vi "Recursive find VIs.vi"(8 "error in (no error)":errorcluster, 11 "Project Items":refnum<vi>[](array[refnum])) -> (0 "error out":errorcluster, 3 "VIs":set{path}(c389))   [LabVIEW 2020, in "Coverage Report.lvclass"]
uses:
  Coverage Report.lvclass
  a1401d1e-ec1c-4a27-9029-e4c0d22f2509.vi
  Coverage Report.lvclass/Coverage Report.ctl
  <vilib>/Astemes/LUnit/Test Case.lvclass
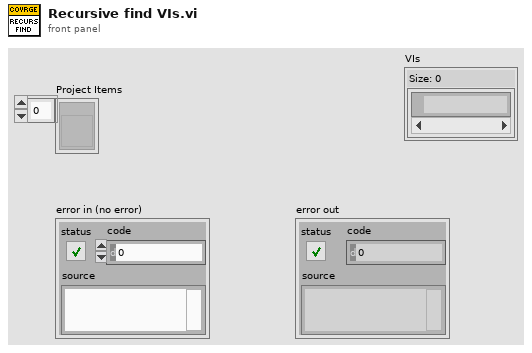
[diagram p1: front panel]
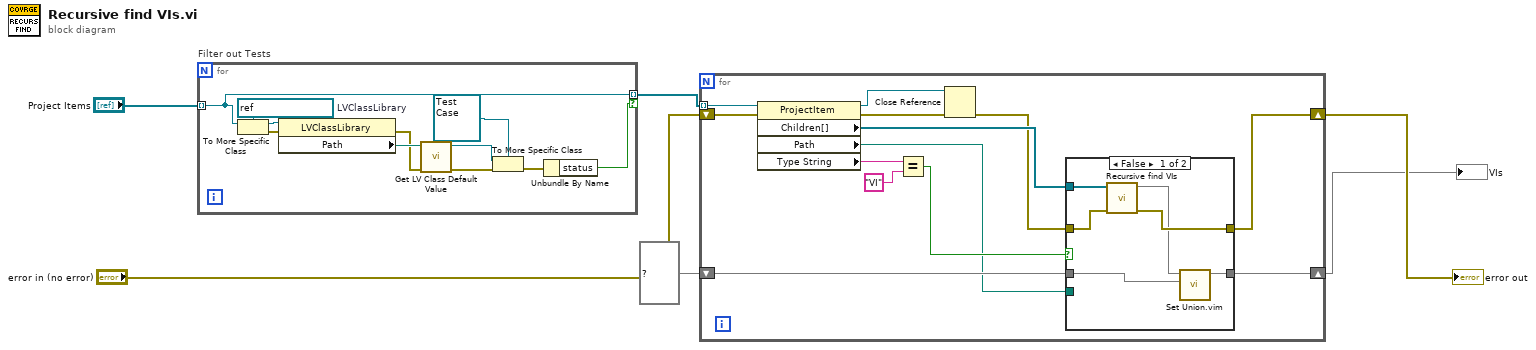
[diagram p0: block diagram]
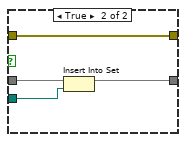
[diagram p2: hidden frame]
diagram:
  n1 = for "Filter out Tests" {
    tunnel: "Project Items" -> [w9] mode=indexing
    tunnel: [w9] -> w1 mode=indexing if=w8
    w17 = refnum<vi> refnum  # LVClassLibrary
    n2 = To More Specific Class(target class=w17, reference=w9) -> (specific class reference=w16:refnum<vi>, error out=w15:errorcluster)  [unwired: 1 in]
    n3 = property class="LVClassLibrary"(reference=w16, error in=w15) -> (error out=w13:errorcluster, "Path"=w14:path)  [unwired: 1 out]
    n4 = call <vilib>:"Get LV Class Default Value.vi"("error in (no error)"=w13, "class path"=w14) -> ("error out"=w12:errorcluster, "object"=w11:refnum<class>)  [unwired: 8 in]
    n5 = To More Specific Class(target class=refnum<class "Test Case.lvclass"> refnum ("LUnit Test Case In"), reference=w11, error in=w12) -> (error out=w10:errorcluster)  [unwired: 1 out]
    n6 = Unbundle By Name(w10) -> ("status"=w8:bool)
  }
  n7 = for {
    tunnel: w1 -> [w27] mode=indexing
    shift-right: [w21] -> w6
    shift-left: "error in (no error)" -> [w26]
    shift-right: [w19] -> w4
    shift-left: set{path} {} ("VIs") -> [w20]
    n8 = property class="ProjectItem"(reference=w27, error in=w26) -> (reference out=w24:refnum<vi>, error out=w25:errorcluster, "Children[]"=w23:refnum<vi>[], "Path"=w18:path, "Type String"=w30:string)
    n9 = Equal?(x=w30, y="VI") -> (x = y?=w28:bool)
    n10 = Close Reference(reference=w24, error in (no error)=w25) -> (error out=w22:errorcluster)
    n11 = case shown="False" w28 {
      tunnel: w23 -> [w36 _]
      tunnel: [w31 w39] -> w19
      tunnel: w22 -> [w35 w40]
      tunnel: [w34 w40] -> w21
      tunnel: w20 -> [w32 w38]
      tunnel: w18 -> [_ w37]
      frame False {
        n12 = call "Recursive find VIs.vi"("error in (no error)"=w35, "Project Items"=w36) -> ("error out"=w34:errorcluster, "VIs"=w33:set{path})  [unwired: 8 in]
        n13 = call "Set Union.vim"("set 2"=w32, "set 1"=w33) -> ("union"=w31:set{path})  [unwired: 9 in]
      }
      frame True {
        n14 = Insert Into Set(10:w37, 11:w38) -> (3:w39:set{path})  [unwired: 1 out]
      }
    }
  }
  "error out" <- w6
  "VIs" <- w4
